vi "RW All ECAT.vi"(2 "R/W Case":T27, 7 "RT Data in":T1={"Device ref"=0, "Scan Period (uSec)"=10000, "Device Channels"={"Status"={"BD Refs"=[], "Length"=0, "FIFO Index"=0, "Data"=[]}, "Command"={"BD Refs"=[], "Data"=[], "Length"=0, "FIFO Index"=0}}, "Local Chassis"=[], "EtherCAT Masters"=[], "Async"={"Status"=refnum, "Command"=refnum, "Input FIFO"=refnum, "Input FIFO buffer"=[], "Output FIFO"=refnum, "Output FIFO buffer"=[], "Async VI Ref"=refnum}, "ECAT Reconfig"={"Reconfig Module Found"=FALSE, "VI Ref"=refnum, "Status"=refnum}, "Device Error"={"status"=FALSE, "code"=0, "source"=""}, "DeviceName"="", "PCLSync?"=FALSE} {"Device Channels"."Status"."BD Refs"."Data Reference" format="%.0x"; "Device Channels"."Command"."BD Refs"."Data Reference" format="%.0x"; "Local Chassis"."FPGA"."VS ref" format="%.0x"; "Local Chassis"."RSI Modules"."VS ref" format="%.0x"; "Local Chassis"."VS ref" format="%.0x"; "Device ref" format="%.0x"; "EtherCAT Masters"."Generic EtherCAT Slaves"."VS ref" format="%.0x"; "EtherCAT Masters"."VS ref" format="%.0x"; "EtherCAT Masters"."EtherCAT Slaves"."FPGA"."VS ref" format="%.0x"; "EtherCAT Masters"."EtherCAT Slaves"."RSI Modules"."VS ref" format="%.0x"; "EtherCAT Masters"."EtherCAT Slaves"."VS ref" format="%.0x"}) -> (8 "RT Data out":T1={"Device ref"=0, "Scan Period (uSec)"=10000, "Device Channels"={"Status"={"BD Refs"=[], "Length"=0, "FIFO Index"=0, "Data"=[]}, "Command"={"BD Refs"=[], "Data"=[], "Length"=0, "FIFO Index"=0}}, "Local Chassis"=[], "EtherCAT Masters"=[], "Async"={"Status"=refnum, "Command"=refnum, "Input FIFO"=refnum, "Input FIFO buffer"=[], "Output FIFO"=refnum, "Output FIFO buffer"=[], "Async VI Ref"=refnum}, "ECAT Reconfig"={"Reconfig Module Found"=FALSE, "VI Ref"=refnum, "Status"=refnum}, "Device Error"={"status"=FALSE, "code"=0, "source"=""}, "DeviceName"="", "PCLSync?"=FALSE} {"Device Channels"."Status"."BD Refs"."Data Reference" format="%.0x"; "Device Channels"."Command"."BD Refs"."Data Reference" format="%.0x"; "Local Chassis"."FPGA"."VS ref" format="%.0x"; "Local Chassis"."RSI Modules"."VS ref" format="%.0x"; "Local Chassis"."VS ref" format="%.0x"; "Device ref" format="%.0x"; "EtherCAT Masters"."Generic EtherCAT Slaves"."VS ref" format="%.0x"; "EtherCAT Masters"."VS ref" format="%.0x"; "EtherCAT Masters"."EtherCAT Slaves"."FPGA"."VS ref" format="%.0x"; "EtherCAT Masters"."EtherCAT Slaves"."RSI Modules"."VS ref" format="%.0x"; "EtherCAT Masters"."EtherCAT Slaves"."VS ref" format="%.0x"})   [LabVIEW 2015, in "Scan Engine Custom Device.lvlib"]
uses:
  Scan Engine Custom Device.lvlib
  Type Defs/RW Case.ctl
  Type Defs/RT Data.ctl
  <vilib>/NI Veristand/Custom Device API/Custom Device Item Ref.ctl
  Type Defs/Device Channels.ctl
  Type Defs/Output Data.ctl
  <vilib>/NI Veristand/Custom Device API/Block Data Reference.ctl
  <vilib>/NI Veristand/Custom Device API/Data Reference.ctl
  Type Defs/Input Data.ctl
  Type Defs/Local Chassis Data.ctl
  Type Defs/RSI Module Data.ctl
  Type Defs/Open Module IOVs.ctl
  Modules.lvlibp/RSI Module/RSI Module.lvclass
  Modules.lvlibp/RSI Module/Module Models.ctl
  Modules.lvlibp/RSI Module/Channel Type.ctl
  Type Defs/Module Config Data.ctl
  Type Defs/Mixed IO.ctl
  Type Defs/FPGA Data.ctl
  Type Defs/UDV Data.ctl
  Type Defs/UDV Data Type.ctl
  Type Defs/FXP Config.ctl
  Type Defs/Mod Size Indexes.ctl
  Type Defs/EtherCAT Master Data.ctl
  Type Defs/EtherCAT Slave Data.ctl
  Type Defs/Generic ECAT Slave RT-Data-Array.ctl
  Type Defs/Generic ECAT Slave Data Cluster.ctl
  Type Defs/Generic ECAT Slave IOV Cluster.ctl
  Type Defs/Async Data.ctl
  Type Defs/Async Status.ctl
  Type Defs/Async State.ctl
  Type Defs/Async Command.ctl
  Type Defs/ECAT Reconfig Data.ctl
  Type Defs/ECAT Reconfig Status.ctl
  Type Defs/ECAT Reconfig State.ctl
  RW Mods.vi
  RW UDVs.vi
  Read ECAT VARs.vi
  Write ECAT VARs.vi
  Read All Input Module Sizes.vi
  Read All Mixed Module Sizes.vi
  Write Module.vi
  Check Module Config.vi
  Read UDVs.vi
  Write UDVs.vi
  Scanned Read - UDV.vi
  <vilib>/NI Veristand/Custom Device API/NI VeriStand - Set Channel Values by Block Data Reference.vi
  Scanned Write - UDV.vi
  <vilib>/NI Veristand/Custom Device API/NI VeriStand - Get Channel Values by Block Data Reference.vi
  Read Input Modules at Indexes.vi
  Read Mixed Modules at Indexes.vi
  Scanned Write - Module.vi
  Read Input Module.vi
  Read Mixed Module.vi
  Scanned Read - Input Module.vi
  Scanned Read - Mixed Module.vi
  <vilib>/NI Veristand/Custom Device API/Global Data Refs.vi
  Launch Local Reconfig.vi
  <vilib>/NI Veristand/Custom Device API/Custom Device API.lvlib
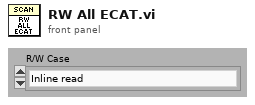
[diagram p1: front panel]
types:
  T1 = typedef "Scan Engine Custom Device.lvlib/RT Data.ctl" = cluster{"Device ref":T2, "Scan Period (uSec)":u32, "Device Channels":T3, "Local Chassis":T8[], "EtherCAT Masters":T20[], "Async":T25, "ECAT Reconfig":T26, "Device Error":errorcluster, "DeviceName":string, "PCLSync?":bool}
  T2 = typedef "Custom Device API.lvlib/Custom Device Item Ref.ctl" = u64
  T3 = typedef "Scan Engine Custom Device.lvlib/Device Channels.ctl" = cluster{"Status":T4, "Command":T7}
  T4 = typedef "Scan Engine Custom Device.lvlib/Output Data.ctl" = cluster{"BD Refs":T5[], "Length":i32, "FIFO Index":i32, "Data":dbl[]}
  T5 = typedef "Custom Device API.lvlib/Block Data Reference.ctl" = cluster{"Data Reference":T6, "Offset":u64, "Length":u64}
  T6 = typedef "Custom Device API.lvlib/Data Reference.ctl" = i32
  T7 = typedef "Scan Engine Custom Device.lvlib/Input Data.ctl" = cluster{"BD Refs":T5[], "Data":dbl[], "Length":i32, "FIFO Index":i32}
  T8 = typedef "Scan Engine Custom Device.lvlib/Local Chassis Data.ctl" = cluster{"VS ref":T2, "RSI Modules":T9[], "FPGA":T15[], "Input Mod Size Idxs":T19, "Output Modules":i32[], "MixedIO Mod Size Idxs":T19}
  T9 = typedef "Scan Engine Custom Device.lvlib/RSI Module Data.ctl" = cluster{"VS ref":T2, "IOV ref":refnum<k21>, "Open Mod refs":T10, "Module DVR":refnum<data-value>, "Slot":u32, "Model":T11, "Channel Type":T12, "EtherCAT?":bool, "CDInput Data":T7, "CDOutput Data":T4, "Module Config Data":T13, "Mixed IO":T14}
  T10 = typedef "Scan Engine Custom Device.lvlib/Open Module IOVs.ctl" = cluster{"Analog Read":refnum<k21>, "Digital Read":refnum<k21>, "Analog Write":refnum<k21>, "Digital Write":refnum<k21>}
  T11 = typedef "Modules.lvlibp/RSI Module.lvclass/Module Models.ctl" = enum16{"Empty", "NI 9201", "NI 9203", "NI 9205", "NI 9206", "NI 9207", "NI 9208", "NI 9211", "NI 9213", "NI 9214", "NI 9215", "NI 9217", "NI 9219", "NI 9221", "NI 9225", "NI 9227", "NI 9229", "NI 9233", "NI 9234", "NI 9235", "NI 9236", "NI 9237", "NI 9239", "NI 9263", "NI 9264", "NI 9265", "NI 9269", "NI 9375", "NI 9401", "NI 9402", "NI 9403", "NI 9411", "NI 9421", "NI 9422", "NI 9423", "NI 9425", "NI 9426", "NI 9435", "NI 9472", "NI 9474", "NI 9475", "NI 9476", "NI 9477", "NI 9478", "NI 9481", "NI 9482", "NI 9485"}
  T12 = typedef "Modules.lvlibp/RSI Module.lvclass/Channel Type.ctl" = enum16{"Analog", "Digital"}
  T13 = typedef "Scan Engine Custom Device.lvlib/Module Config Data.ctl" = cluster{"Configurable?":bool, "Config Block Data Refs":T5[], "Config Data DVR":refnum<data-value>, "Previous Values":dbl[], "Local Reconfig VI Ref":refnum<vi>}
  T14 = typedef "Scan Engine Custom Device.lvlib/Mixed IO.ctl" = cluster{"Input Channel Indices":i32[], "Input Buffer":dbl[]}
  T15 = typedef "Scan Engine Custom Device.lvlib/FPGA Data.ctl" = cluster{"VS ref":T2, "IOV ref":refnum<k21>, "FPGA Target":enum16{"Local", "EtherCAT"}, "Product Code":u32, "Bitfile Signature":string, "Bitfile Path (RT)":path, "FPGA Session":u32, "Input Data":T7, "Output Data":T4, "UDVs":cluster{"From FPGA":T16[], "To FPGA":T16[]}}
  T16 = typedef "Scan Engine Custom Device.lvlib/UDV Data.ctl" = cluster{"VS ref":T2, "IOV Ref":refnum<k21>, "Name":string, "UDV Data Type":T17, "Supported Type?":bool, "FXP Config":T18, "FXP VI Ref":refnum<vi>}
  T17 = typedef "Scan Engine Custom Device.lvlib/UDV Data Type.ctl" = enum16{"Boolean", "Fixed Point", "Int8", "Int16", "Int32", "Int64", "U32 Bit Field", "UInt8", "UInt16", "UInt32", "UInt64", "Other"}
  T18 = typedef "Scan Engine Custom Device.lvlib/FXP Config.ctl" = cluster{"signed":bool, "size":u32, "integersize":i32}
  T19 = typedef "Scan Engine Custom Device.lvlib/Mod Size Indexes.ctl" = cluster{"4":i32[], "8":i32[], "16":i32[], "32":i32[], "other":i32[]}
  T20 = typedef "Scan Engine Custom Device.lvlib/EtherCAT Master Data.ctl" = cluster{"VS ref":T2, "IOV ref":refnum<k21>, "Master ID":u32, "Cyclic Data Bandwidth":u32, "EtherCAT Slaves":T21[], "Generic EtherCAT Slaves":T22}
  T21 = typedef "Scan Engine Custom Device.lvlib/EtherCAT Slave Data.ctl" = cluster{"VS ref":T2, "IOV ref":refnum<k21>, "Position Address":u16, "RSI Modules":T9[], "FPGA":T15[], "Input Mod Size Idxs":T19, "Output Modules":i32[], "MixedIO Mod Size Idxs":T19}
  T22 = typedef "Scan Engine Custom Device.lvlib/Generic ECAT Slave RT-Data-Array.ctl" = T23[]
  T23 = typedef "Scan Engine Custom Device.lvlib/Generic ECAT Slave Data Cluster.ctl" = cluster{"VS ref":T2, "IOV ref":refnum<k21>, "Position Address":u16, "I/O Imput Vars ":T24[], "I/O Output Vars":T24[], "I/O Input Data":T7, "I/O Output Data":T4}
  T24 = typedef "Scan Engine Custom Device.lvlib/Generic ECAT Slave IOV Cluster.ctl" = cluster{"VS ref":T2, "IOV Ref":refnum<k21>, "Name":string, "UDV Data Type":T17}
  T25 = typedef "Scan Engine Custom Device.lvlib/Async Data.ctl" = cluster{"Status":refnum<queue>, "Command":refnum<queue>, "Input FIFO":refnum<k33>, "Input FIFO buffer":dbl[], "Output FIFO":refnum<k33>, "Output FIFO buffer":dbl[], "Async VI Ref":refnum<vi>}
  T26 = typedef "Scan Engine Custom Device.lvlib/ECAT Reconfig Data.ctl" = cluster{"Reconfig Module Found":bool, "VI Ref":refnum<vi>, "Status":refnum<queue>}
  T27 = typedef "Scan Engine Custom Device.lvlib/RW Case.ctl" = enum16{"Inline read", "Inline write", "Async - Inline loop read", "Async - Inline loop write", "Async loop (read/write)"}
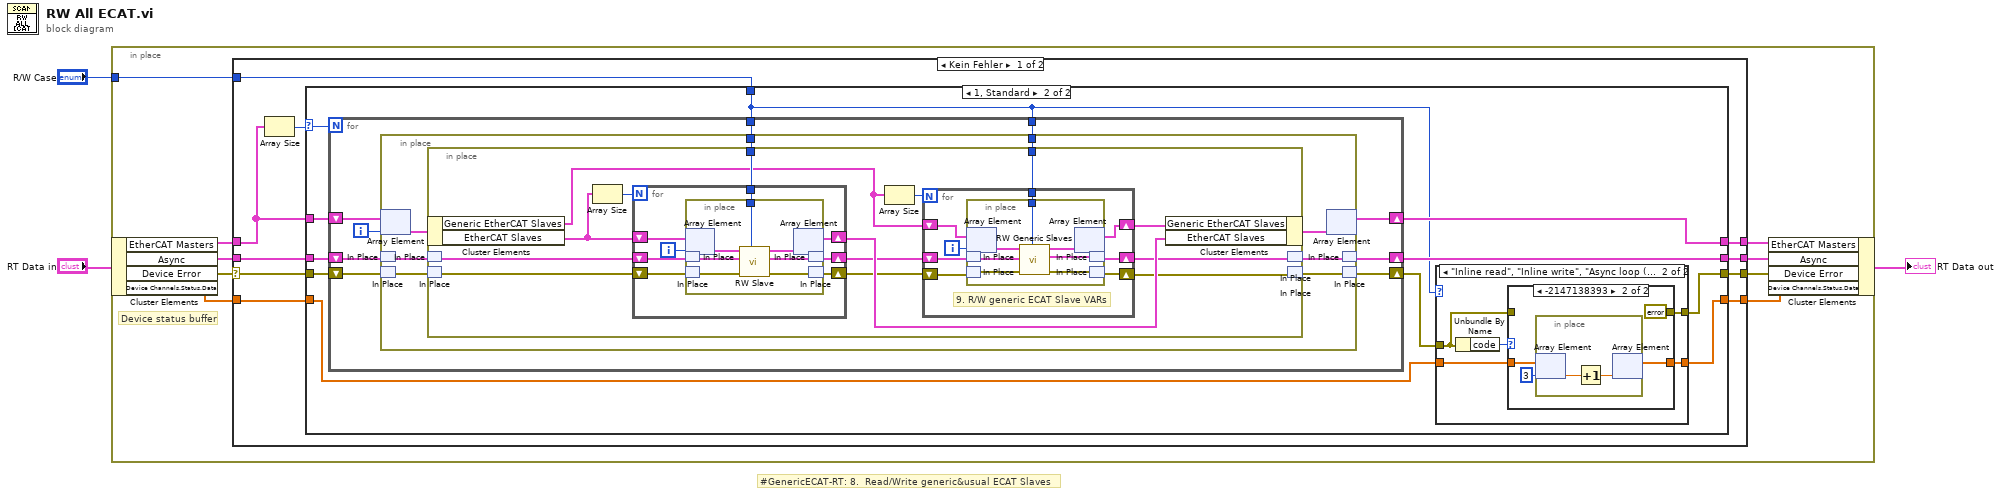
[diagram p0: block diagram]
diagram:
  # "#GenericECAT-RT: 8.  Read/Write generic&usual ECAT Slaves"
  n1 = in-place {
    in-place-border: "R/W Case" -> [w6]
    # "Device status buffer"
    n2 = in-place-cluster #1("RT Data in") -> ("EtherCAT Masters"=w7:T20[], "Async"=w9:T25, "Device Error"=w12:errorcluster, "Device Channels.Status.Data"=w5:dbl[])
    n3 = case shown="Kein Fehler" w12 {
      selector: w12 -> [w20 w117]
      tunnel: [w15 w117] -> w11
      tunnel: [w18 w116] -> w10
      tunnel: w9 -> [w21 w116]
      tunnel: [w19 w115] -> w8
      tunnel: w7 -> [w22 w115]
      tunnel: w6 -> [w17 _]
      tunnel: w5 -> [w16 w114]
      tunnel: [w13 w114] -> w4
      frame No Error {
        n4 = Array Size(array=w22) -> (size(s)=w14:i32)
        n5 = case shown="1, Standard" w14 {
          selector: w14 -> [_ w30]
          tunnel: w22 -> [w26 w37]
          tunnel: w21 -> [w25 w36]
          tunnel: w20 -> [w24 w35]
          tunnel: [w26 w34] -> w19
          tunnel: [w25 w33] -> w18
          tunnel: w17 -> [_ w27]
          tunnel: w16 -> [w23 w29]
          tunnel: [w24 w31] -> w15
          tunnel: [w23 w28] -> w13
          frame 0 {
          }
          frame 1, Default {
            n6 = for {
              N: w30 -> [_]
              shift-right: [w55] -> w32
              shift-left: w35 -> [w56]
              shift-right: [w59] -> w34
              shift-left: w37 -> [w61]
              shift-right: [w57] -> w33
              shift-left: w36 -> [w58]
              tunnel: w27 -> [w54]
              tunnel: w27 -> [w53]
              i -> [w60]
              n7 = in-place {
                in-place-border: w54 -> [w63]
                in-place-border: w53 -> [w62]
                n8 = in-place-array #2(w61, w60) -> (w69:T20)
                n9 = in-place-match #3(w58) -> (w67:T25)
                n10 = in-place-match #4(w56) -> (w65:errorcluster)
                n11 = in-place {
                  in-place-border: w63 -> [w80]
                  in-place-border: w62 -> [w73]
                  n12 = in-place-cluster #5(w69) -> ("Generic EtherCAT Slaves"=w72:T22, "EtherCAT Slaves"=w79:T21[])
                  n13 = in-place-match #6(w67) -> (w82:T25)
                  n14 = in-place-match #7(w65) -> (w81:errorcluster)
                  n15 = Array Size(array=w79) -> (size(s)=w83:i32)
                  n16 = for {
                    N: w83 -> [_]
                    shift-right: [w104] -> w78
                    shift-left: w79 -> [w106]
                    shift-right: [w99] -> w76
                    shift-left: w81 -> [w100]
                    shift-right: [w102] -> w77
                    shift-left: w82 -> [w103]
                    tunnel: w80 -> [w101]
                    i -> [w105]
                    n17 = in-place {
                      in-place-border: w101 -> [w110]
                      n18 = in-place-array #8(w106, w105) -> (w107:T21)
                      n19 = in-place-match #9(w103) -> (w112:T25)
                      n20 = in-place-match #10(w100) -> (w109:errorcluster)
                      n21 = call "RW Slave.vi"("R/W Case"=w110, "error in (no error)"=w109, "Async in"=w112, "Slave in"=w107) -> ("error out"=w108:errorcluster, "Async out"=w111:T25, "Slave out"=w113:T21)  [unwired: 5 in]
                      n22 = in-place-array #8(w113) -> (w104:T21[])  [unwired: 1 out]
                      n23 = in-place-match #9(w111) -> (w102:T25)
                      n24 = in-place-match #10(w108) -> (w99:errorcluster)
                    }
                  }
                  n25 = Array Size(array=w72) -> (size(s)=w70:i32)
                  n26 = for {
                    N: w70 -> [_]
                    shift-right: [w87] -> w75
                    shift-left: w76 -> [w88]
                    shift-right: [w86] -> w74
                    shift-left: w77 -> [w89]
                    shift-right: [w90] -> w71
                    shift-left: w72 -> [w91]
                    tunnel: w73 -> [w85]
                    i -> [w84]
                    # "9. R/W generic ECAT Slave VARs"
                    n27 = in-place {
                      in-place-border: w85 -> [w96]
                      n28 = in-place-array #11(w91, w84) -> (w98:T23)
                      n29 = in-place-match #12(w89) -> (w93:T25)
                      n30 = in-place-match #13(w88) -> (w95:errorcluster)
                      n31 = call "RW Generic Slaves.vi"("R/W Case"=w96, "error in (no error)"=w95, "Async in"=w93, "Generic ECAT Slaves in"=w98) -> ("error out"=w94:errorcluster, "Async out"=w92:T25, "Generic ECAT Slaves out"=w97:T23)  [unwired: 5 in]
                      n32 = in-place-array #11(w97) -> (w90:T22)  [unwired: 1 out]
                      n33 = in-place-match #12(w92) -> (w86:T25)
                      n34 = in-place-match #13(w94) -> (w87:errorcluster)
                    }
                  }
                  n35 = in-place-cluster #5("Generic EtherCAT Slaves"=w71, "EtherCAT Slaves"=w78) -> (w68:T20)
                  n36 = in-place-match #6(w74) -> (w66:T25)
                  n37 = in-place-match #7(w75) -> (w64:errorcluster)
                }
                n38 = in-place-array #2(w68) -> (w59:T20[])  [unwired: 1 out]
                n39 = in-place-match #3(w66) -> (w57:T25)
                n40 = in-place-match #4(w64) -> (w55:errorcluster)
              }
            }
            n41 = case shown="\"Inline read\", \"Inline write\", \"Async loop (read/write)\"" w27 {
              tunnel: w32 -> [w39 w43]
              tunnel: [w39 w42] -> w31
              tunnel: w29 -> [w38 w41]
              tunnel: [w38 w40] -> w28
              frame Default {
              }
              frame "Inline read", "Inline write", "Async loop (read/write)" {
                n42 = Unbundle By Name(w43) -> ("code"=w44:i32)
                n43 = case shown="-2147138393" w44 {
                  tunnel: w43 -> [w46 _]
                  tunnel: [w46 errorcluster {"status"=FALSE, "code"=0, "source"=""} ("error IO")] -> w42
                  tunnel: [w45 w47] -> w40
                  tunnel: w41 -> [w45 w49]
                  frame 0, Default {
                  }
                  frame -2147138393 {
                    n44 = in-place {
                      n45 = in-place-array #14(w49, 3) -> (w52:dbl)
                      n46 = Increment(x=w52) -> (x+1=w51:dbl)
                      n47 = in-place-array #14(w51) -> (w47:dbl[])  [unwired: 1 out]
                    }
                  }
                }
              }
            }
          }
        }
      }
      frame Error {
      }
    }
    n48 = in-place-cluster #1("EtherCAT Masters"=w8, "Async"=w10, "Device Error"=w11, "Device Channels.Status.Data"=w4) -> (→"RT Data out":T1)
  }
